vi "SEM_RESULT.vi"(4 "RO":bool, 8 "error in":errorcluster {"code" format="%.0x"}, 11 "Session In":refnum<visa-resource-name>="TCPIP0::K-N90X0A-00005.local::hislip0::INSTR") -> (0 "error out":errorcluster {"code" format="%.0x"}, 3 "Session Out":refnum<visa-resource-name>, 5 "RefFreq(MHz)":dbl)   [LabVIEW 2018]
panel:
  in  "read":string=":MEAS:SEM 1?"
  in  "write":string="INIT:SEM"
  out "string":string
  in  "Timeout":u32=3000
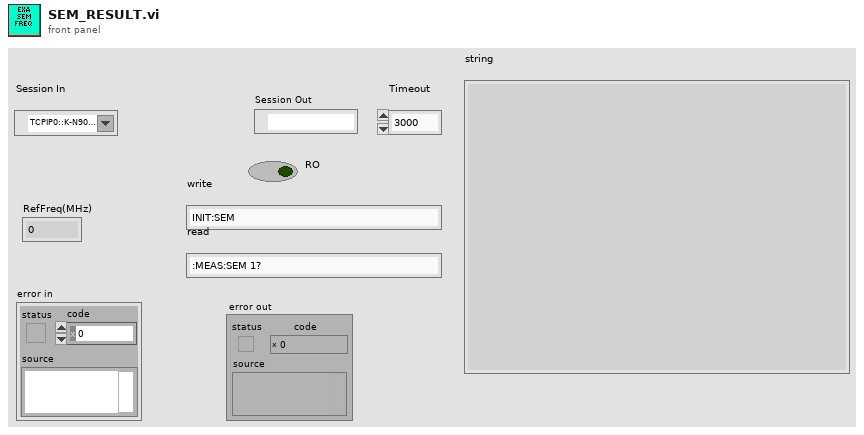
[diagram p1: front panel]
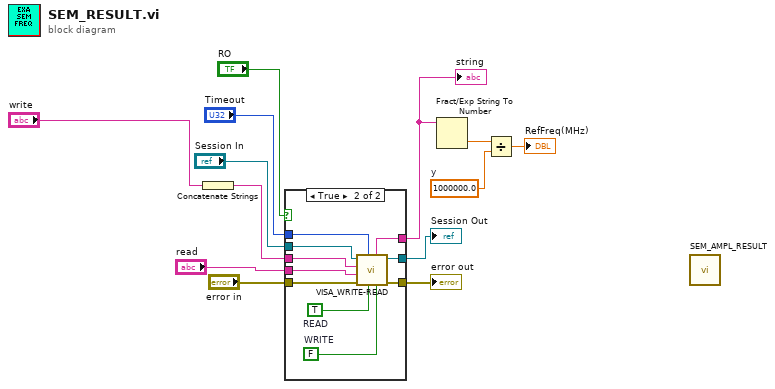
[diagram p0: block diagram]
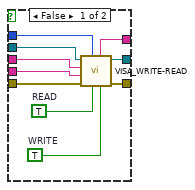
[diagram p2: hidden frame]
diagram:
  w4 = 1000000.0  # y
  n1 = Concatenate Strings("write") -> (w10:string)
  n2 = case shown="True" "RO" {
    tunnel: "error in" -> [w23 w33]
    tunnel: [w22 w32] -> w12
    tunnel: w10 -> [w21 w31]
    tunnel: "read" -> [w20 w30]
    tunnel: "Session In" -> [w19 w29]
    tunnel: [w18 w28] -> w7
    tunnel: [w17 w27] -> w1
    tunnel: "Timeout" -> [w16 w26]
    frame False {
      w14 = TRUE  # WRITE
      w15 = TRUE  # READ
      n3 = call "VISA_WRITE-READ.vi"("WRITE"=w14, "READ"=w15, "Timeout"=w16, "error in"=w23, "Rcmd"=w20, "Wcmd"=w21, "Session In"=w19) -> ("error out"=w22:errorcluster, "Session Out"=w18:refnum<visa-resource-name>, "Out"=w17:string)  [unwired: 2 in]
    }
    frame True {
      w24 = FALSE  # WRITE
      w25 = TRUE  # READ
      n4 = call "VISA_WRITE-READ.vi"("WRITE"=w24, "READ"=w25, "Timeout"=w26, "error in"=w33, "Rcmd"=w30, "Wcmd"=w31, "Session In"=w29) -> ("error out"=w32:errorcluster, "Session Out"=w28:refnum<visa-resource-name>, "Out"=w27:string)  [unwired: 2 in]
    }
  }
  "error out" <- w12
  "Session Out" <- w7
  "string" <- w1
  n5 = Fract/Exp String To Number(string=w1) -> (number=w5:dbl)  [unwired: 3 in, 1 out]
  n6 = Divide(x=w5, y=w4) -> (x/y=→"RefFreq(MHz)":dbl)
  n7 = call "SEM_AMPL_RESULT.vi"() -> ()  [unwired: 11 in, 5 out]
